vi "Add PV - String Array.vi"(5 "is read only? (F)":bool, 6 "initial timestamp":timestamp, 7 "PV name":string, 8 "error in (no error)":errorcluster, 10 "initial value":string[](array[string]), 11 "Server in":refnum<class "Server.lvclass">) -> (0 "error out":errorcluster, 3 "Server out":refnum<class "Server.lvclass">)   [LabVIEW 2020, in "PV Access.lvlib" / "PVA Server.lvlib" / "Server.lvclass"]
uses:
  Server.lvclass
  Server.lvclass/Server.ctl
  PV Data/NT Scalar/NT Scalar.lvclass
  Source/Source.lvclass
  PV Data/PV Data.lvlib
  PV Data/NT Scalar/Create - String Array.vi
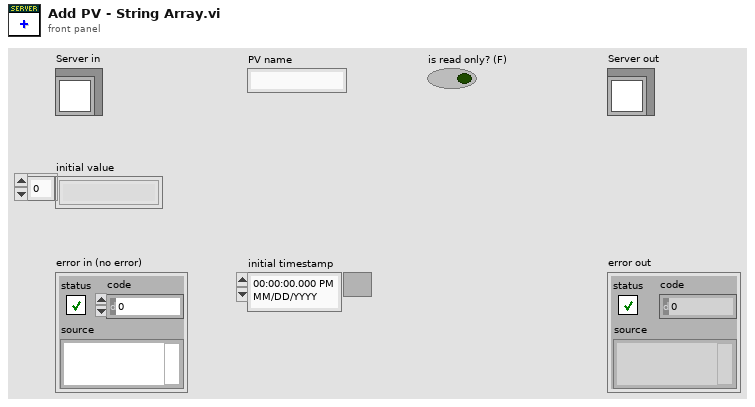
[diagram p1: front panel]
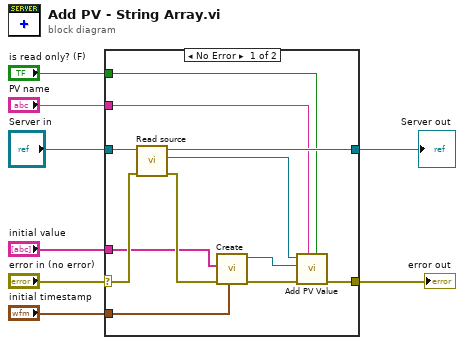
[diagram p0: block diagram]
diagram:
  n1 = case shown="No Error" "error in (no error)" {
    selector: "error in (no error)" -> [w16 w22]
    tunnel: [w15 w22] -> w7
    tunnel: [w19 w21] -> w5
    tunnel: "Server in" -> [w20 w21]
    tunnel: "PV name" -> [w17 _]
    tunnel: "initial value" -> [w11 _]
    tunnel: "initial timestamp" -> [w10 _]
    tunnel: "is read only? (F)" -> [w9 _]
    frame No Error {
      n2 = call "Read source.vi"("error in (no error)"=w16, "Server in"=w20) -> ("error out"=w14:errorcluster, "Source"=w18:refnum<class "Source.lvclass">, "Server out"=w19:refnum<class "Server.lvclass">)  [unwired: 7 in]
      n3 = call-poly "Create.vi"("timestamp in"=w10, "error in (no error)"=w14, "value in"=w11) -> ("error out"=w13:errorcluster, "NT Scalar out"=w12:refnum<class "NT Scalar.lvclass">)  [unwired: 7 in]
      n4 = call "Add PV Value.vi"("is read only? (F)"=w9, "PV name"=w17, "error in"=w13, "NT Base in"=w12, "Source in"=w18) -> ("error out"=w15:errorcluster)  [unwired: 4 in, 2 out]
    }
    frame Error {
    }
  }
  "error out" <- w7
  "Server out" <- w5
